vi "Validate_Destination_Core.vi"(8 "error in (no error)":errorcluster, 10 "Destination":refnum<class "AB_Destination.lvclass">, 11 "AB_Source in":refnum<class "AB_Source.lvclass">) -> (0 "error out":errorcluster, 2 "valid":bool, 3 "AB_Source out":refnum<class "AB_Source.lvclass">)   [LabVIEW 2020, in "AB_Source.lvclass"]
uses:
  <vilib>/AppBuilder/AB_Classes/Source/AB_Source.lvclass
  <vilib>/AppBuilder/AB_Classes/Destination/AB_Destination.lvclass
  <vilib>/AppBuilder/AB_Classes/Source/AB_Source.lvclass/AB_Source.ctl
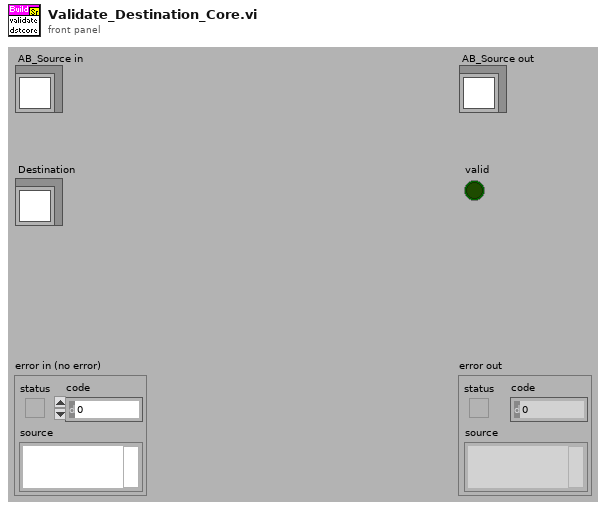
[diagram p1: front panel]
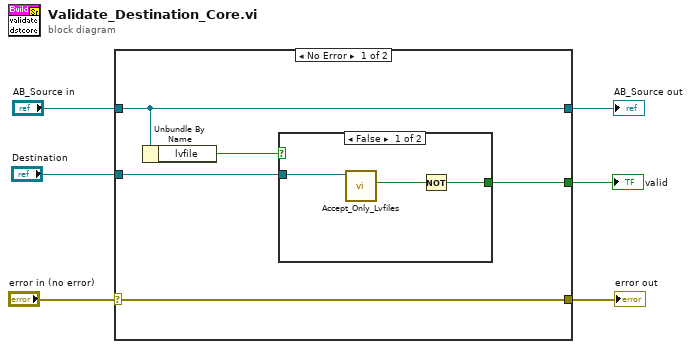
[diagram p0: block diagram]
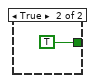
[diagram p2: hidden frame]
diagram:
  n1 = case shown="No Error" "error in (no error)" {
    selector: "error in (no error)" -> [w11 w17]
    tunnel: [w11 w17] -> w5
    tunnel: [w8 w16] -> w3
    tunnel: "AB_Source in" -> [w8 w16]
    tunnel: "Destination" -> [w10 _]
    tunnel: [w9 _] -> w1
    frame No Error {
      n2 = Unbundle By Name(w8) -> ("lvfile"=w7:bool)
      n3 = case shown="False" w7 {
        tunnel: w10 -> [w14 _]
        tunnel: [w12 TRUE] -> w9
        frame False {
          n4 = call-dynamic "Accept_Only_Lvfiles.vi"("AB_Destination in"=w14) -> ("onlyLVfiles"=w13:bool)  [unwired: 8 in, 2 out]
          n5 = Not(x=w13) -> (.not. x?=w12:bool)
        }
        frame True {
        }
      }
    }
    frame Error {
    }
  }
  "error out" <- w5
  "AB_Source out" <- w3
  "valid" <- w1
